vi "CSM Watchdog Thread.vi"(11 "Watchdog Queue":refnum<queue>) -> ()   [LabVIEW 2017, in "CSM Watchdog.lvlib"]
doc: "The CSM Watchdog thread is used to ensure that all asynchronously started CSM modules can exit normally after the main program exits.\n\n\n> [!NOTE] <b>CSM WatchDog Implementation Principle</b>\n>\n> When a LabVIEW VI exits, it automatically releases all handle resources such as queues and events. Therefore, you can create a WatchDog thread that monitors a queue resource created by the main program VI. When this queue resource is released after the main VI exits, the WatchDog thread is triggered to send \"Macro: Exit\" to any CSM modules that have not yet exited, ensuring they exit normally.\n\n\n-- <b>Controls</b> --\n- <b>Watchdog Queue</b>: Watchdog queue resource."
uses:
  CSM Watchdog.lvlib
  AdvanceAPI/CSM - Filter Messages to Non-Existing Modules.vi
  Communicable State Machine.lvlib
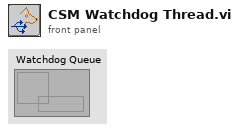
[diagram p1: front panel]
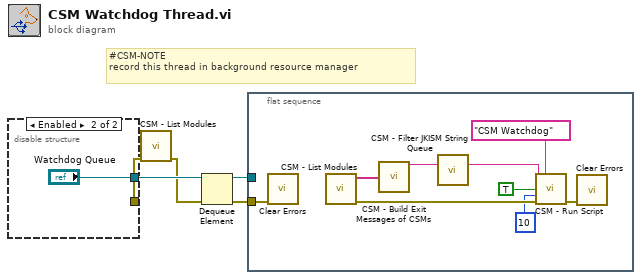
[diagram p0: block diagram]
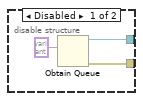
[diagram p2: hidden frame]
diagram:
  # "#CSM-NOTE\nrecord this thread in background resource manager"
  n1 = disable-structure shown="Enabled" {
    disable-tunnel: [w7 _] -> w2
    disable-tunnel: [w6 "Watchdog Queue"] -> w5
    frame Disabled {
      n2 = Obtain Queue(element data type=variant) -> (queue out=w6:refnum<queue>, error out=w7:errorcluster)  [unwired: 4 in, 1 out]
    }
    frame Enabled {
    }
  }
  n3 = call "CSM - List Modules.vi"("Error In"=w2) -> ("error out"=w1:errorcluster)  [unwired: 9 in, 1 out]
  n4 = Dequeue Element(queue=w5, error in (no error)=w1) -> (queue out=w3:refnum<queue>, error out=w4:errorcluster)  [unwired: 1 in, 2 out]
  n5 = flat-sequence {
    tunnel: w4 -> [w13]
    tunnel: w3 -> [_]
    frame #0 {
      n6 = call <vilib>:"Clear Errors.vi"("error in (no error)"=w13) -> ()  [unwired: 5 in, 2 out]
      n7 = call "CSM - List Modules.vi"() -> ("error out"=w16:errorcluster, "Module Names"=w17:string[])  [unwired: 10 in]
      n8 = call "CSM - Build Exit Messages of CSMs.vi"("CSMs"=w17) -> ("States"=w18:string)  [unwired: 14 in]
      n9 = call-poly "CSM - Filter JKISM String Queue.vi"("States In"=w18) -> ("States Out"=w15:string)  [unwired: 14 in]
      n10 = call "CSM - Run Script.vi"("CSM Scripts"=w15, "Current Module (\"\" to Generate an ID)"="CSM Watchdog" ("Current Module(\"\" to generate a ID)"), "Continue If Error? (F)"=TRUE ("Continue If Error?(F)"), "Wait (5000ms)"=10 ("Wait(5000ms)"), "error in (no error)"=w16) -> ("error out"=w14:errorcluster)  [unwired: 8 in, 2 out]
      n11 = call <vilib>:"Clear Errors.vi"("error in (no error)"=w14) -> ()  [unwired: 5 in, 2 out]
    }
  }
